vi "GPIO for ADC.vi"(8 "error in (no error)":errorcluster, 10 "AnalogIn":refnum<class "AI.lvclass">, 11 "Session in":refnum<class "Session.lvclass">) -> (0 "error out":errorcluster, 2 "GPIO":refnum<class "GPIO.lvclass">, 3 "Session out":refnum<class "Session.lvclass">)   [LabVIEW 2020, in "CTI.lvlib" / "Session.lvclass"]
uses:
  Session.lvclass
  Session.lvclass/Session.ctl
  AI/AI.lvclass
  GPIO/GPIO.lvclass
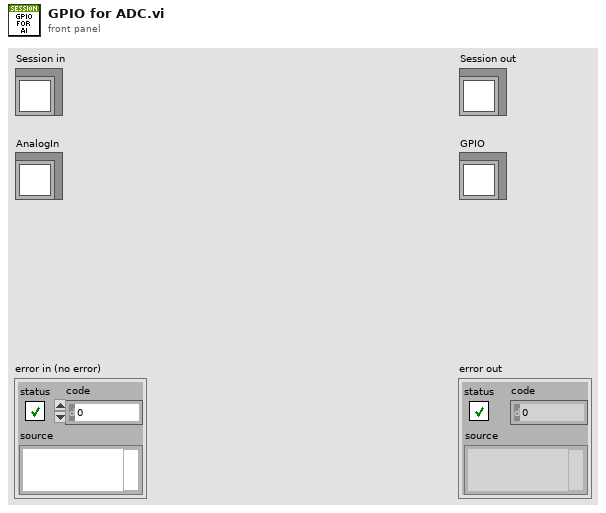
[diagram p1: front panel]
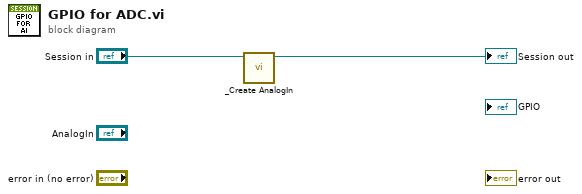
[diagram p0: block diagram]
diagram:
  n1 = call "_Create AnalogIn.vi"("Session in"="Session in") -> ("Session out"=→"Session out":refnum<class "Session.lvclass">)  [unwired: 8 in, 2 out]
